vi "ExFileReadNConvertToU16.vi"() -> ()   [LabVIEW 2010]
panel:
  in  "Full File Name":path
  in  "?":bool
  in  "FileType":u32=67371008
  out "error out":errorcluster
  in  "error in (no error)":errorcluster
  # "ExReadFileNconvertToU16.vi\nThis example will read in a file of the\nselected data type and display as u16 frame.\nWhen finished viewing data, make sure to\nuse the STOP button to close the display."
  # "File Types:\nSPE = 67371008\nTIF   = 67174400\nPMI  = 67436544"
  # "Browse match pattern is set to *.spe.  Modify this if different file type is needed."
  # "This will properly close\nthe image and\ndeallocate memory."
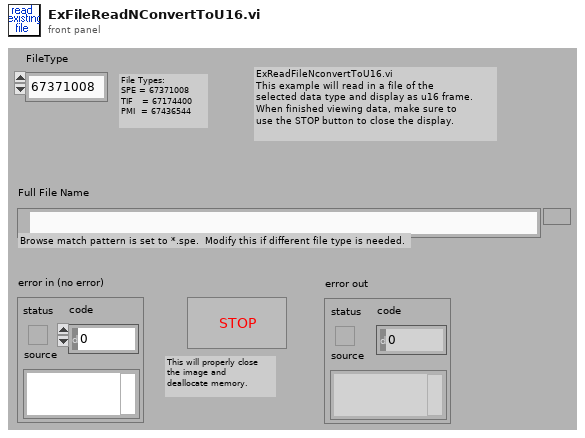
[diagram p1: front panel]
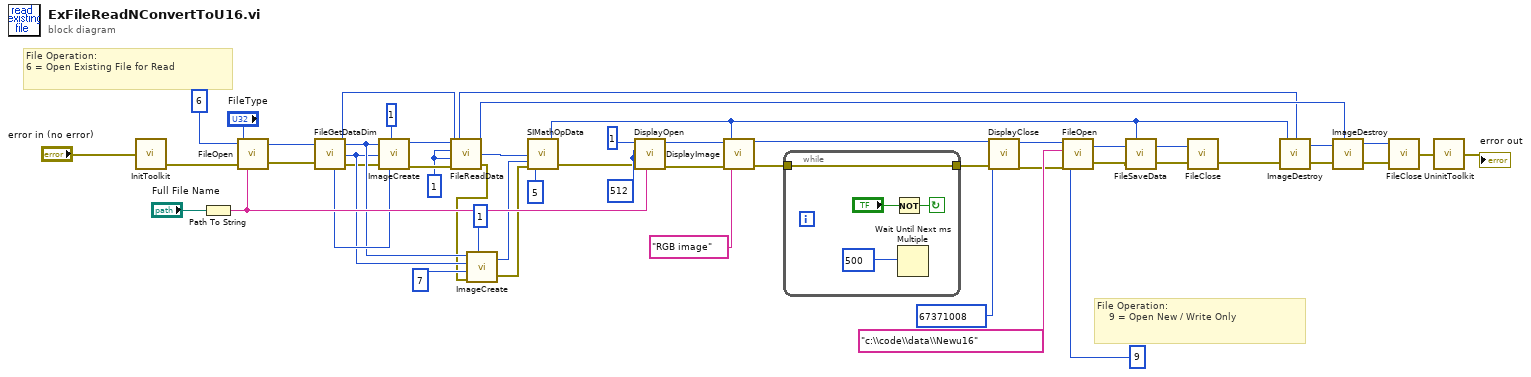
[diagram p0: block diagram]
diagram:
  w33 = 1
  w41 = 512
  # "File Operation:\n    9 = Open New / Write Only"
  # "File Operation:\n6 = Open Existing File for Read"
  n1 = call <userlib>:"InitToolkit.vi"("error in"="error in (no error)") -> ("error out"=w46:errorcluster)
  n2 = Path To String(path="Full File Name") -> (string=w36:string)
  n3 = call <userlib>:"FileOpen.vi"("error in"=w46, "File Operations"=u32 6 ("File Operation"), "FileName"=w36, "File Type"="FileType") -> ("error out"=w44:errorcluster, "File Handle"=w43:u32)
  n4 = call <userlib>:"FileGetDataDim.vi"("File Handle"=w43, "error in"=w44) -> ("Data Type"=w23:u32, "File Handle"=w35:u32, "X dim"=w22:u32, "Y dim"=w21:u32, "error out"=w17:errorcluster)  [unwired: 1 out]
  n5 = call <userlib>:"ImageCreate.vi"("X dimension"=w22, "Y dimension"=w21, "Data Type"=w23, "error in"=w17, "Number Of Frames"=1) -> ("Image Handle"=w25:u32, "error out"=w34:errorcluster)
  n6 = call <userlib>:"FileReadData.vi"("File Handle"=w35, "Start Frame"=w33, "End Frame"=w33, "error in"=w34, "Image Handle"=w25) -> ("File Handle"=w32:u32, "Image Handle"=w14:u32, "error out"=w18:errorcluster)
  n7 = call <userlib>:"ImageCreate.vi"("X dimension"=w22, "Y dimension"=w21, "Data Type"=7, "error in"=w18, "Number Of Frames"=1) -> ("Image Handle"=w15:u32, "error out"=w16:errorcluster)
  n8 = call <userlib>:"SIMathOpData.vi"("error in (no error)"=w16, "Operation"=5, "Result Handle"=w15, "Data Handle"=w14) -> ("error out"=w12:errorcluster, "Result Handle"=w4:u32)
  n9 = call <userlib>:"DisplayOpen.vi"("Display Title"=w36, "error in"=w12, "Display Height"=w41, "Display Width"=w41, "Display Type"=1) -> ("error out"=w31:errorcluster, "Display Handle"=w30:u32)  [unwired: 1 in]
  n10 = call <userlib>:"DisplayImage.vi"("error in"=w31, "Title"="RGB image", "Image Handle"=w4, "Display Handle"=w30) -> ("error out"=w24:errorcluster, "Display Handle"=w29:u32)
  n11 = while {
    tunnel: w24 -> [w49]
    tunnel: [w49] -> w3
    stop <- w51 continue-if-true
    n12 = Not(x="?") -> (.not. x?=w51:bool)
    n13 = Wait Until Next ms Multiple(millisecond multiple=500) -> ()  [unwired: 1 out]
  }
  n14 = call <userlib>:"DisplayClose.vi"("error in"=w3, "Display Handle"=w29) -> ("error out"=w2:errorcluster)
  n15 = call <userlib>:"FileOpen.vi"("error in"=w2, "File Operations"=9, "FileName"="c:\\code\\data\\Newu16", "File Type"=67371008) -> ("error out"=w11:errorcluster, "File Handle"=w9:u32)
  n16 = call <userlib>:"FileSaveData.vi"("error in"=w11, "Image Handle"=w4, "File Handle"=w9) -> ("error out"=w10:errorcluster, "File Handle"=w8:u32)
  n17 = call <userlib>:"FileClose.vi"("error in"=w10, "File Handle"=w8) -> ("error out"=w1:errorcluster)
  n18 = call <userlib>:"ImageDestroy.vi"("error in"=w1, "Data handle"=w4) -> ("error out"=w28:errorcluster)
  n19 = call <userlib>:"ImageDestroy.vi"("error in"=w28, "Data handle"=w25) -> ("error out"=w27:errorcluster)
  n20 = call <userlib>:"FileClose.vi"("error in"=w27, "File Handle"=w32) -> ("error out"=w39:errorcluster)
  n21 = call <userlib>:"UninitToolkit.vi"("error in"=w39) -> ("error out"=→"error out":errorcluster)
